vi "SEA-9811_ReceiverLoopback_ReverseU8Bitorder.vi"(11 "U8 in":u8) -> (3 "Bit reversed U8 out":u8)   [LabVIEW 2017]
doc: "Reverses the bitorder of an U8 value.\n\nCopyright (c) 2013-2019 S.E.A. Datentechnik GmbH, Germany"
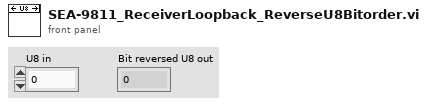
[diagram p1: front panel]
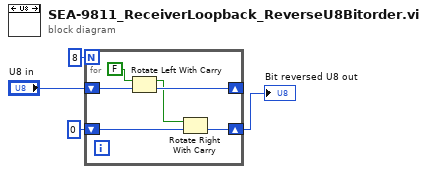
[diagram p0: block diagram]
diagram:
  n1 = for {
    N: 8 -> [_]
    shift-right: [w7] -> _
    shift-left: "U8 in" -> [w10]
    shift-right: [w8] -> w4
    shift-left: u8 0 -> [w9]
    n2 = Rotate Left With Carry(2:w10, 3:FALSE ("carry")) -> (0:w7:u8, 1:w6:bool)
    n3 = Rotate Right With Carry(2:w9, 3:w6) -> (0:w8:u8)  [unwired: 1 out]
  }
  "Bit reversed U8 out" <- w4
